vi "S2C_M2p5942_Proc_Channels.vi"(7 "Local?":bool, 8 "Error In":errorcluster, 10 "Command":string, 11 "JSON String":string) -> (0 "Error Out":errorcluster, 3 "Response":variant)   [LabVIEW 2024]
uses:
  S2C_M2p5942_Proc_Globals.vi
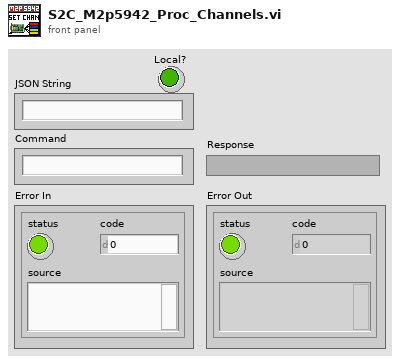
[diagram p1: front panel]
types:
  T1 = cluster{"CH0 Enable":bool, "CH0 Range":u16, "CH0 Term":u16, "CH0 Type":u16, "CH0 Offset":i32, "CH1 Enable":bool, "CH1 Range":u16, "CH1 Term":u16, "CH1 Type":u16, "CH1 Offset":i32, "CH2 Enable":bool, "CH2 Range":u16, "CH2 Term":u16, "CH2 Type":u16, "CH2 Offset":i32, "CH3 Enable":bool, "CH3 Range":u16, "CH3 Term":u16, "CH3 Type":u16, "CH3 Offset":i32}
  T2 = cluster{"AI Channels":i32, "AI Ranges":i32, "Input Ranges (mV)":i32[], "Programmable Offset":i32, "Termination Available":bool, "SE/Diff switchable":bool, "Offset in per cent/mV":bool, "Offset Calibration":bool, "Gain Calibration":bool, "Offset with open inputs":bool, "AI Range Strings[]":string[], "Bit Resolution":i32, "AC Coupling available":bool, "BW Limit available":bool, "AI Path count":i32}
  T3 = cluster{"CH0 Enable":bool, "CH0 Range":u16, "CH0 Term":u16, "CH0 Type":u16, "CH0 Offset":i32}
  T4 = cluster{"CH1 Enable":bool, "CH1 Range":u16, "CH1 Term":u16, "CH1 Type":u16, "CH1 Offset":i32}
  T5 = cluster{"CH2 Enable":bool, "CH2 Range":u16, "CH2 Term":u16, "CH2 Type":u16, "CH2 Offset":i32}
  T6 = cluster{"CH3 Enable":bool, "CH3 Range":u16, "CH3 Term":u16, "CH3 Type":u16, "CH3 Offset":i32}
  T7 = cluster{"CH3 Enable":bool, "CH3 Range":u16, "CH3 Term":u16, "CH3 Type":u16, "CH3 Offset":i32}[]
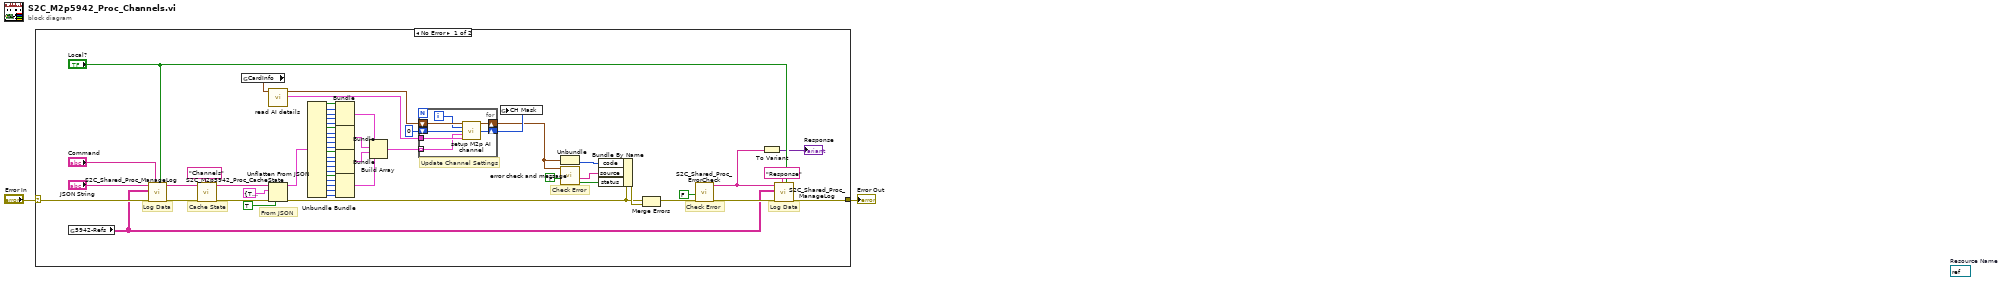
[diagram p0: block diagram]
diagram:
  (unwired) refnum<visa-resource-name> refnum  # Resource Name
  n1 = case shown="No Error" "Error In" {
    selector: "Error In" -> [w58 w67]
    tunnel: [w56 w67] -> w1
    frame No Error {
      # "Check Error"
      # "Update Channel Settings"
      # "Check Error"
      # "Cache State"
      # "Log Data"
      # "Log Data"
      # "From JSON"
      n2 = global read "S2C_M2p5942_Proc_Globals.vi" "5942-Refs"() -> (w46:string[][])
      n3 = call "S2C_Shared_Proc_ManageLog.vi"("Local?"="Local?", "Command"="Command", "Error In"=w58, "Refs"=w46, "Data In"="JSON String") -> ("Error Out"=w54:errorcluster, "Data Out"=w53:string)  [unwired: 5 in]
      n4 = call "S2C_M2p5942_Proc_CacheState.vi"("Label"="Channels", "Error In"=w54, "Data In"=w53) -> ("Error Out"=w51:errorcluster, "Data Out"=w52:string)  [unwired: 7 in]
      n5 = global read "S2C_M2p5942_Proc_Globals.vi" "CardInfo"() -> (w44:cluster{"Card Handle":u64, "Error Code":u32})
      n6 = call "read AI details.vi"("Card Info In"=w44) -> ("AI Details"=w12:T2, "Card Info Out"=w11:cluster{"Card Handle":u64, "Error Code":u32})  [unwired: 5 in]
      n7 = Unflatten From JSON(JSON string=w52, type and defaults=T1 {"CH0 Enable"=TRUE, "CH0 Range"=2, "CH0 Term"=0, "CH0 Type"=0, "CH0 Offset"=0, "CH1 Enable"=TRUE, "CH1 Range"=2, "CH1 Term"=0, "CH1 Type"=0, "CH1 Offset"=0, "CH2 Enable"=TRUE, "CH2 Range"=2, "CH2 Term"=0, "CH2 Type"=0, "CH2 Offset"=0, "CH3 Enable"=TRUE, "CH3 Range"=2, "CH3 Term"=0, "CH3 Type"=0, "CH3 Offset"=0} ("Channels"), default null elements? (F)=TRUE, error in (no error)=w51) -> (value=w18:T1, error out=w4:errorcluster)  [unwired: 3 in]
      n8 = Unbundle(w18) -> ("CH0 Enable"=w38:bool, "CH0 Range"=w34:u16, "CH0 Term"=w35:u16, "CH0 Type"=w36:u16, "CH0 Offset"=w37:i32, "CH1 Enable"=w33:bool, "CH1 Range"=w30:u16, "CH1 Term"=w29:u16, "CH1 Type"=w28:u16, "CH1 Offset"=w27:i32, "CH2 Enable"=w32:bool, "CH2 Range"=w26:u16, "CH2 Term"=w25:u16, "CH2 Type"=w24:u16, "CH2 Offset"=w23:i32, "CH3 Enable"=w31:bool, "CH3 Range"=w22:u16, "CH3 Term"=w21:u16, "CH3 Type"=w20:u16, "CH3 Offset"=w19:i32)
      n9 = Bundle("CH0 Enable"=w38, "CH0 Range"=w34, "CH0 Term"=w35, "CH0 Type"=w36, "CH0 Offset"=w37) -> (w17:T3)  [unwired: 1 in]
      n10 = Bundle("CH1 Enable"=w33, "CH1 Range"=w30, "CH1 Term"=w29, "CH1 Type"=w28, "CH1 Offset"=w27) -> (w16:T4)  [unwired: 1 in]
      n11 = Bundle("CH2 Enable"=w32, "CH2 Range"=w26, "CH2 Term"=w25, "CH2 Type"=w24, "CH2 Offset"=w23) -> (w14:T5)  [unwired: 1 in]
      n12 = Bundle("CH3 Enable"=w31, "CH3 Range"=w22, "CH3 Term"=w21, "CH3 Type"=w20, "CH3 Offset"=w19) -> (w15:T6)  [unwired: 1 in]
      n13 = Build Array(w17, w16, w14, w15) -> (w13:T7)
      n14 = for {
        tunnel: w12 -> [w65]
        tunnel: w13 -> [w64] mode=indexing
        shift-right: [w62] -> w42
        shift-left: u32 0 ("Channel MaskOut") -> [w61]
        shift-right: [w60] -> w5
        shift-left: w11 -> [w66]
        i -> [w63]
        n15 = call "setup M2p AI channel.vi"("Card Info In"=w66, "Channel Index"=w63, "Channel Mask In"=w61, "AI Channel"=w64, "AI details"=w65) -> ("Card Info Out"=w60:cluster{"Card Handle":u64, "Error Code":u32}, "Channel MaskOut"=w62:u32)  [unwired: 7 in, 2 out]
      }
      n16 = global write "S2C_M2p5942_Proc_Globals.vi" "CH Mask"(w42) -> ()
      n17 = Unbundle(w5) -> ("Error Code"=w8:u32)  [unwired: 1 out]
      n18 = call "error check and message.vi"("Display Message (true)"=FALSE, "Card Info In"=w5) -> ("Error occurred"=w6:bool, "Error Message"=w7:string)  [unwired: 3 in, 1 out]
      n19 = Bundle By Name(cluster=w4, "code"=w8, "source"=w7, "status"=w6) -> (w10:errorcluster)
      n20 = Merge Errors(w4, w10) -> (w3:errorcluster)
      n21 = call "S2C_Shared_Proc_ErrorCheck.vi"("Error In"=w3, "ExpReply?"=FALSE) -> ("Error Out"=w48:errorcluster, "Status"=w41:string)  [unwired: 8 in]
      n22 = To Variant(anything=w41) -> (Variant=→"Response":variant)
      n23 = call "S2C_Shared_Proc_ManageLog.vi"("Local?"="Local?", "Command"="Response", "Error In"=w48, "Refs"=w46, "Data In"=w41) -> ("Error Out"=w56:errorcluster)  [unwired: 5 in, 1 out]
    }
    frame Error {
    }
  }
  "Error Out" <- w1
